vi "自动ROI转换（T3转T2）.vi"(1 "ROI输入(T3)":T1) -> (0 "ROI输出(T2)":T1)   [LabVIEW 2017]
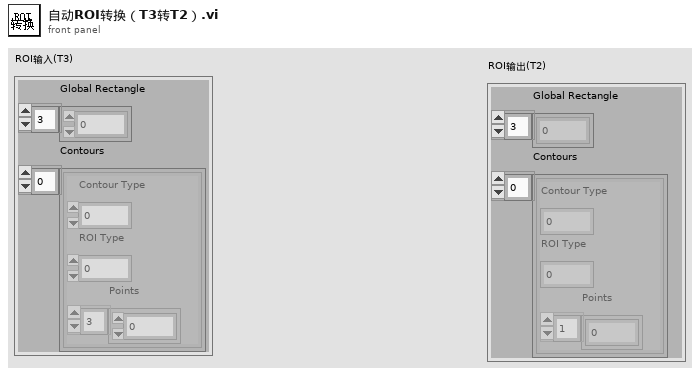
[diagram p1: front panel]
types:
  T1 = cluster{"Global Rectangle":i32[], "Contours":cluster{"Contour Type":u32, "ROI Type":u32, "Points":i32[]}[]}
  T2 = cluster{"Contour Type":u32, "ROI Type":u32, "Points":i32[]}[]
  T3 = cluster{"Contour Type":u32, "ROI Type":u32, "Points":i32[]}
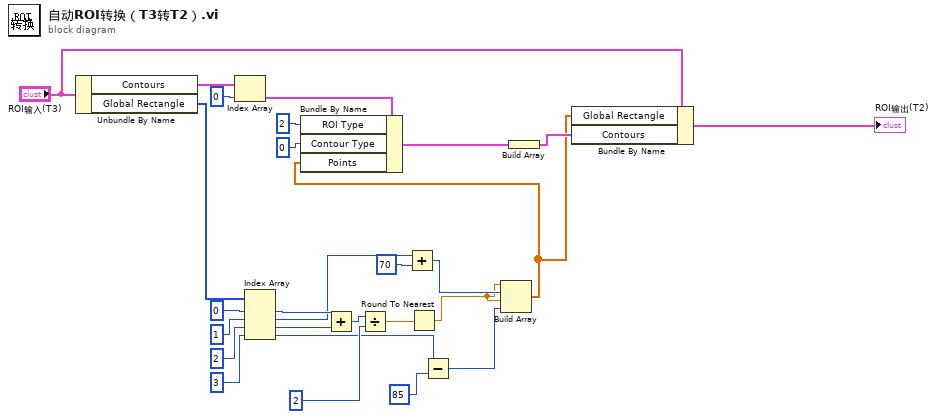
[diagram p0: block diagram]
diagram:
  n1 = Unbundle By Name("ROI输入(T3)") -> ("Contours"=w27:T2, "Global Rectangle"=w22:i32[])
  n2 = Index Array(array=w27, index=0 ("索引")) -> (element=w25:T3)
  n3 = Index Array(array=w22, index #1=u32 0 ("ROI Type"), index #2=u32 1 ("ROI Type"), index #3=u32 2 ("ROI Type"), index #4=u32 3 ("ROI Type")) -> (element #1=w12:i32, element #2=w7:i32, element #3=w11:i32, element #4=w3:i32)
  n4 = Add(x=w12, y=w11) -> (x+y=w10:i32)
  n5 = Divide(x=w10, y=2) -> (x/y=w8:dbl)
  n6 = Add(x=w7, y=70) -> (x+y=w5:i32)
  n7 = Round To Nearest(number=w8) -> (nearest integer value=w1:dbl)
  n8 = Subtract(x=w3, y=85) -> (x-y=w2:i32)
  n9 = Build Array(w1, w5, w1, w2) -> (w14:dbl[])
  n10 = Bundle By Name(cluster=w25, "ROI Type"=u32 2, "Contour Type"=u32 0 ("ROI Type"), "Points"=w14) -> (w17:T3)
  n11 = Build Array(w17) -> (w15:T2)
  n12 = Bundle By Name(cluster="ROI输入(T3)", "Global Rectangle"=w14, "Contours"=w15) -> (→"ROI输出(T2)":T1)
